vi "SDSU_Initialize.vi"(0 "refnum":i32, 5 "Utility Path":path, 7 "Timing Path":path, 9 "Pci Path":path, 11 "error in (no error)":errorcluster, 12 "Memory Parameters":T2, 13 "Database RefNum in":T1) -> (4 "refnum out":i32, 15 "error out":errorcluster)   [LabVIEW 2016]
uses:
  DBSHAND/private/vis/DatabaseHand_RefNum.ctl
panel:
  in  "tryes":i32
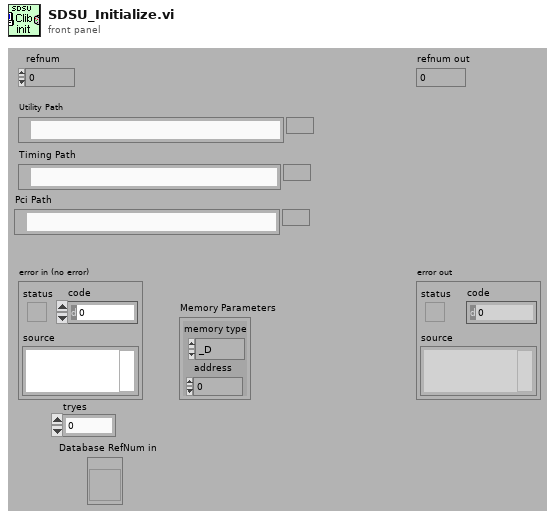
[diagram p1: front panel]
types:
  T1 = typedef "DatabaseHand_RefNum.ctl" = refnum<vi>
  T2 = cluster{"memory type":enum16{"_D", "_P", "_X", "_R", "_Y"}, "address":i32}
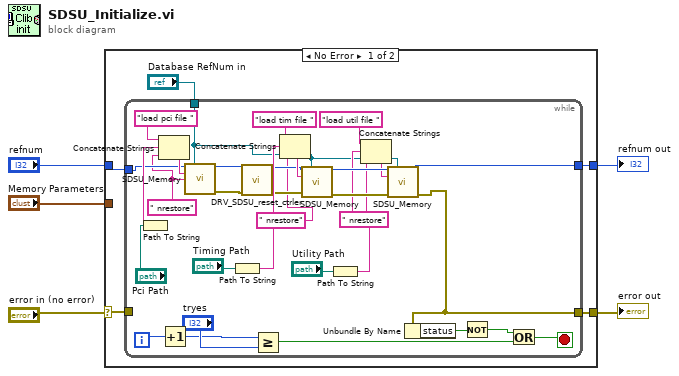
[diagram p0: block diagram]
diagram:
  n1 = case shown="No Error" "error in (no error)" {
    selector: "error in (no error)" -> [w7 w43]
    tunnel: [w9 w43] -> w5
    tunnel: "refnum" -> [w10 w44]
    tunnel: [w8 w44] -> w3
    tunnel: "Memory Parameters" -> [_ _]
    frame No Error {
      n2 = while {
        tunnel: w7 -> [_]
        tunnel: [w40] -> w8
        tunnel: [w37] -> w9
        tunnel: w10 -> [w19]
        tunnel: "Database RefNum in" -> [w14]
        i -> [w34]
        stop <- w38 stop-if-true
        w11 = " nrestore" ("string")
        n3 = Path To String(path="Pci Path") -> (string=w27:string)
        n4 = Concatenate Strings("load pci file ", w27, w11) -> (w26:string)
        n5 = Increment(x=w34) -> (x+1=w32:i32)
        n6 = call "SDSU_Memory.vi"("refnum"=w19, "Database RefNum in"=w14, "Command In"=w26, "physical unit"=w11) -> ("refnum out"=w17:i32, "error out"=w18:errorcluster)  [unwired: 1 in, 9 out]
        n7 = Path To String(path="Timing Path") -> (string=w24:string)
        n8 = call "DRV_SDSU_reset_ctrler.vi"("fd"=w17, "error in (no error)"=w18) -> ("fd out"=w16:i32, "error out"=w15:errorcluster)  [unwired: 12 out]
        n9 = Greater Or Equal?(x=w32, y="tryes") -> (x >= y?=w39:bool)
        n10 = Concatenate Strings("load tim file " ("string"), w24, " nrestore" ("string")) -> (w23:string)
        n11 = call "SDSU_Memory.vi"("refnum"=w16, "Database RefNum in"=w14, "Command In"=w23, "error in (no error)"=w15) -> ("refnum out"=w42:i32, "error out"=w41:errorcluster)  [unwired: 1 in, 9 out]
        n12 = Path To String(path="Utility Path") -> (string=w21:string)
        n13 = Concatenate Strings("load util file " ("string"), w21, " nrestore" ("string")) -> (w20:string)
        n14 = call "SDSU_Memory.vi"("refnum"=w42, "Database RefNum in"=w14, "Command In"=w20, "error in (no error)"=w41) -> ("refnum out"=w40:i32, "error out"=w37:errorcluster)  [unwired: 1 in, 9 out]
        n15 = Unbundle By Name(w37) -> ("status"=w36:bool)
        n16 = Not(x=w36) -> (.not. x?=w35:bool)
        n17 = Or(x=w35, y=w39) -> (x .or. y?=w38:bool)
      }
    }
    frame Error {
    }
  }
  "error out" <- w5
  "refnum out" <- w3
